vi "Lex Number.vi"(8 "error in (no error)":errorcluster, 11 "JSON Lexer in":refnum<class "JSON Lexer.lvclass">) -> (0 "error out":errorcluster, 1 "EOF":bool, 2 "Next State":T1=enum."Value", 3 "JSON Lexer out":refnum<class "JSON Lexer.lvclass">)   [LabVIEW 2019, in "JKI JSON Serialization.lvlib" / "JSON Lexer.lvclass"]
doc: "JKI JSON 1.1.10.37\nTomi Maila - JKI\nCopyright (c) 2017, JKI"
uses:
  JSON Lexer.lvclass
  JSON Lexer States.ctl
  JSON Lexer.lvclass/JSON Lexer.ctl
  Unicode/UTF-8 String/UTF-8 String.lvclass/UTF-8 String.ctl
  Unicode/UTF-8 String/Index Rune as UTF-8 Substring.vi
  Unicode/UTF-8 String/Next Rune As UTF-8 Substring.vi
  Unicode/UTF-8 String/Bytes In Rune.vi
  <vilib>/Utility/error.llb/Error Cluster From Error Code.vi
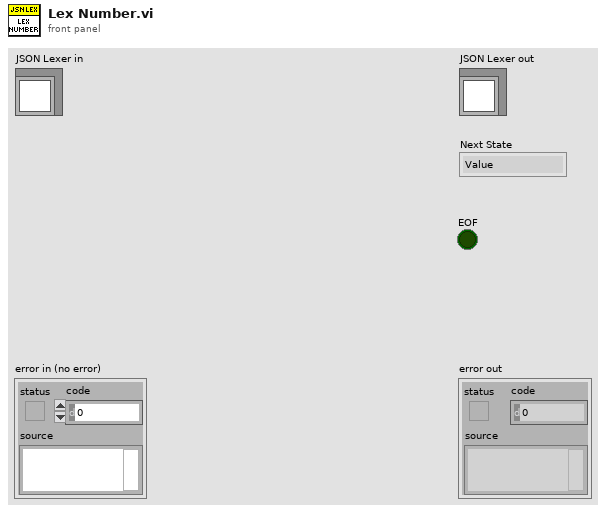
[diagram p1: front panel]
types:
  T1 = typedef "JKI JSON Serialization.lvlib/JSON Lexer.lvclass/JSON Lexer States.ctl" = enum16{"Undefined", "Value", "String", "Numeric", "Number", "Symbol", "Symbolic Number"}
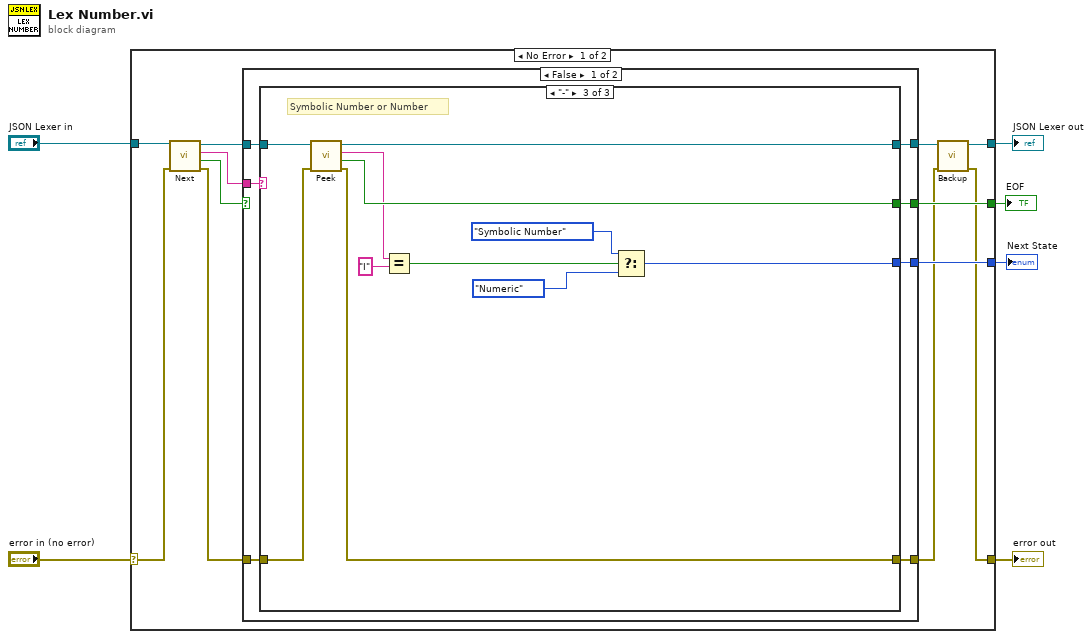
[diagram p0: block diagram]
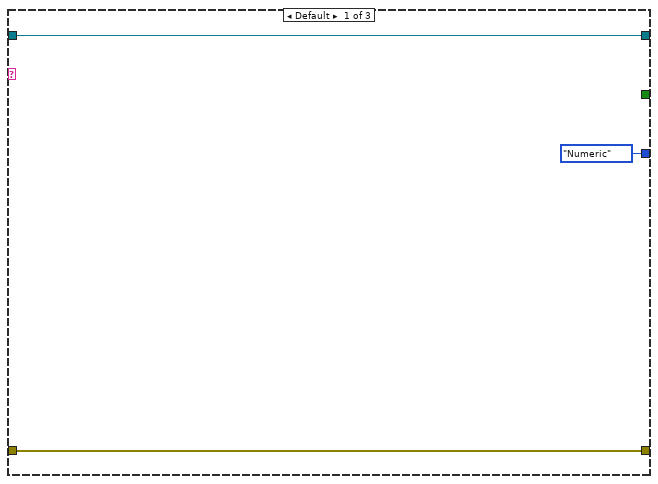
[diagram p2: hidden frame]
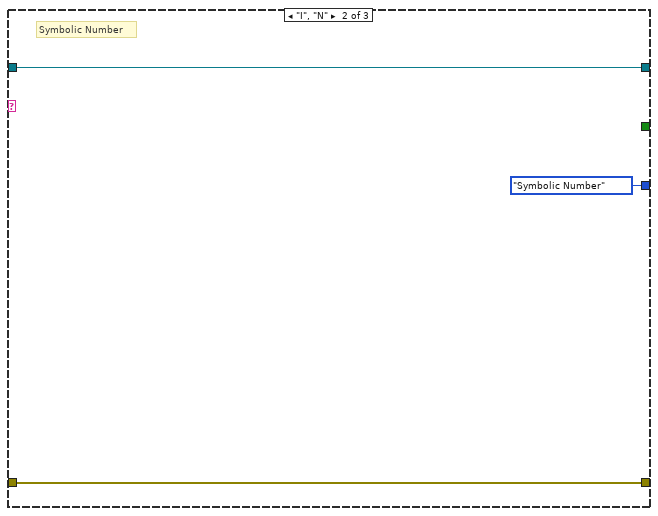
[diagram p3: hidden frame]
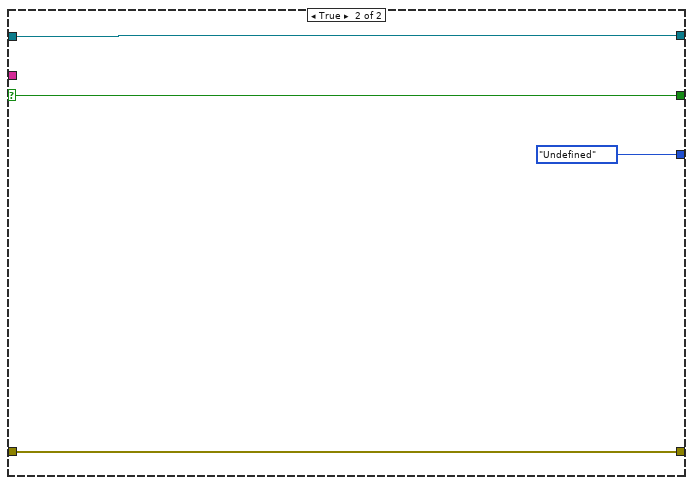
[diagram p4: hidden frame]
diagram:
  n1 = case shown="No Error" "error in (no error)" {
    selector: "error in (no error)" -> [w12 w48]
    tunnel: [w8 w48] -> w5
    tunnel: [w9 w47] -> w3
    tunnel: "JSON Lexer in" -> [w11 w47]
    tunnel: [w14 _] -> w2
    tunnel: [w13 _] -> w1
    frame No Error {
      n2 = call "Next.vi"("error in (no error)"=w12, "JSON Lexer in"=w11) -> ("error out"=w15:errorcluster, "EOF"=w18:bool, "Rune"=w17:string, "JSON Lexer out"=w16:refnum<class "JSON Lexer.lvclass">)  [unwired: 6 in]
      n3 = case shown="False" w18 {
        selector: w18 -> [_ w44]
        tunnel: w17 -> [w23 _]
        tunnel: w16 -> [w25 w46]
        tunnel: w15 -> [w22 w45]
        tunnel: [w21 w45] -> w7
        tunnel: [w24 w46] -> w10
        tunnel: [w20 w44] -> w14
        tunnel: [w19 JSON_Lexer_States."Undefined" ("Next State")] -> w13
        frame False {
          n4 = case shown="\"-\"" w23 {
            tunnel: w25 -> [w28 w30 w42]
            tunnel: [w28 w30 w41] -> w24
            tunnel: w22 -> [w27 w29 w40]
            tunnel: [w27 w29 w39] -> w21
            tunnel: [_ _ w38] -> w20
            tunnel: [JSON_Lexer_States."Numeric" ("f") JSON_Lexer_States."Symbolic Number" ("Next State") w33] -> w19
            frame Default {
            }
            frame "I", "N" {
              # "Symbolic Number"
            }
            frame "-" {
              # "Symbolic Number or Number"
              n5 = call "Peek.vi"("error in (no error)"=w40, "JSON Lexer in"=w42) -> ("error out"=w39:errorcluster, "EOF"=w38:bool, "Rune"=w36:string, "JSON Lexer out"=w41:refnum<class "JSON Lexer.lvclass">)  [unwired: 6 in]
              n6 = Equal?(x=w36, y="I" ("Accepted Runes")) -> (x = y?=w35:bool)
              n7 = Select(t=JSON_Lexer_States."Symbolic Number" ("Next State"), s=w35, f=JSON_Lexer_States."Numeric") -> (s? t:f=w33:T1)
            }
          }
        }
        frame True {
        }
      }
      n8 = call "Backup.vi"("error in (no error)"=w7, "JSON Lexer in"=w10) -> ("error out"=w8:errorcluster, "JSON Lexer out"=w9:refnum<class "JSON Lexer.lvclass">)  [unwired: 8 in]
    }
    frame Error {
    }
  }
  "error out" <- w5
  "JSON Lexer out" <- w3
  "Next State" <- w1
  "EOF" <- w2
